vi "Resistance_measuremetn.vi"() -> ()   [LabVIEW 2015]
panel:
  out "XY Graph 2":cluster{dbl[], dbl[]}(graph)
  in  "Sample 2":refnum<visa-resource-name>
  out "number":dbl
  in  "milliseconds to wait":u32
  in  "VISA resource name 2":refnum<visa-resource-name>
  in  "Sample 1":refnum<visa-resource-name>
  in  "stop":bool
  out "XY Graph":cluster{dbl[], dbl[]}(graph)
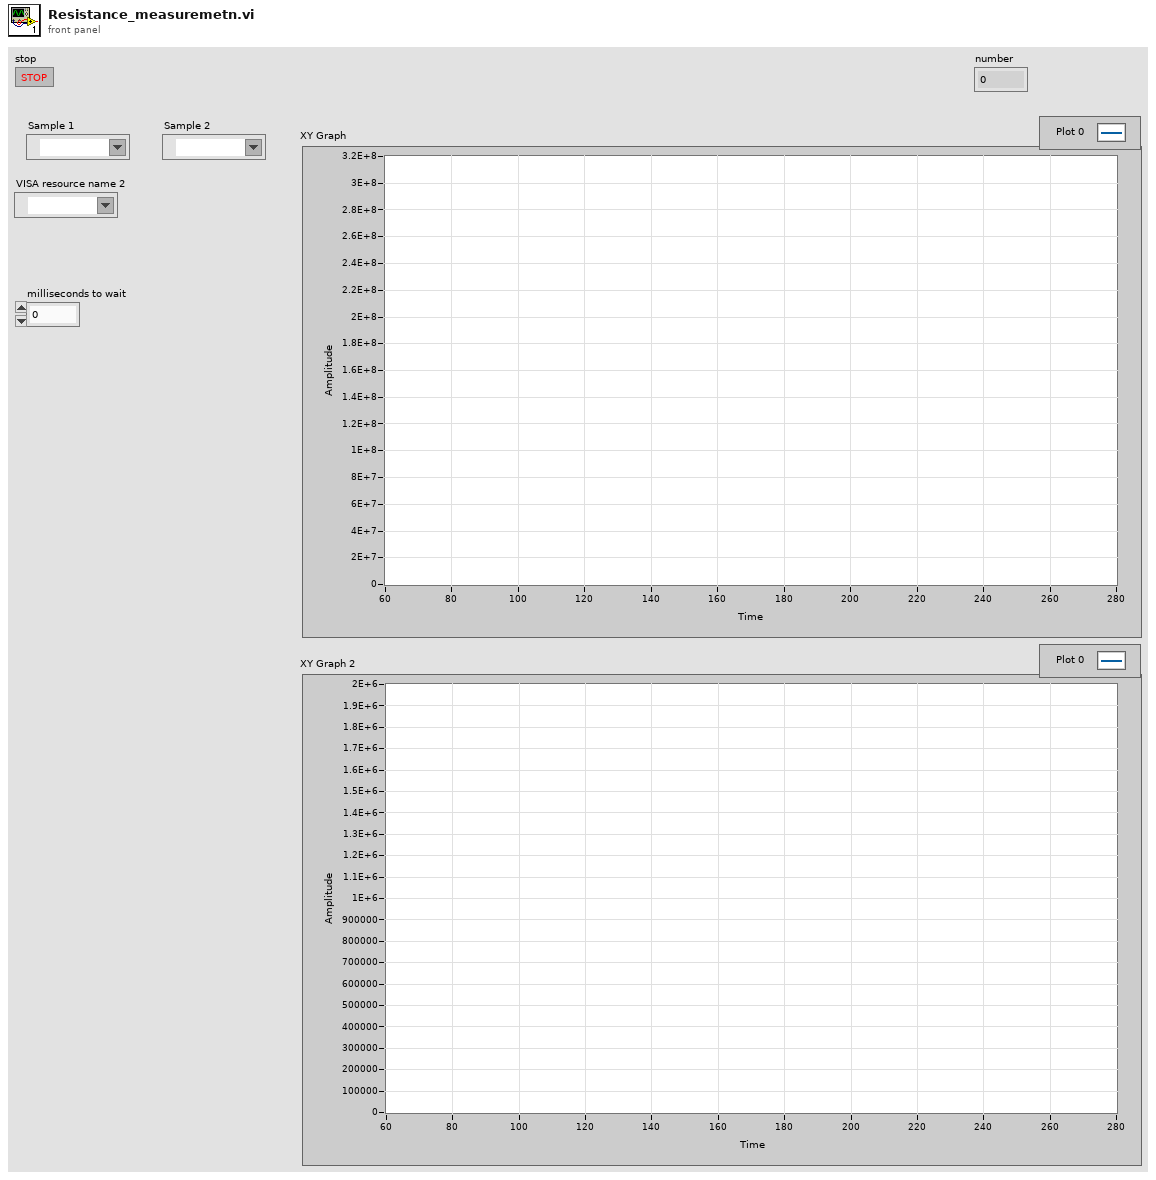
[diagram p1: front panel]
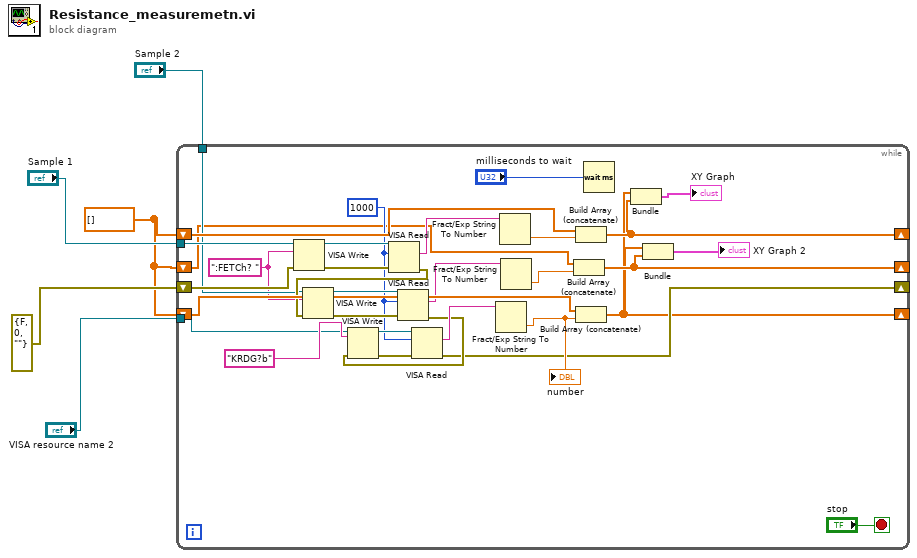
[diagram p0: block diagram]
diagram:
  w1 = dbl[] []
  n1 = while {
    tunnel: "Sample 1" -> [w35]
    tunnel: "VISA resource name 2" -> [w29]
    shift-right: [w7] -> _
    shift-left: w1 -> [w26]
    shift-right: [w23] -> _
    shift-left: w1 -> [w24]
    shift-right: [w17] -> _
    shift-left: errorcluster {"status"=FALSE, "code"=0, "source"=""} ("error out") -> [w16]
    tunnel: "Sample 2" -> [w15]
    shift-right: [w8] -> _
    shift-left: w1 -> [w9]
    stop <- "stop" stop-if-true
    w13 = ":FETCh? " ("write buffer")
    w12 = u32 1000 ("byte count")
    n2 = VISA Write(VISA resource name=w35, write buffer=w13, error in (no error)=w16) -> (VISA resource name out=w34:refnum<visa-resource-name>, error out=w36:errorcluster)  [unwired: 1 out]
    n3 = VISA Read(VISA resource name=w34, byte count=w12, error in (no error)=w36) -> (read buffer=w33:string, error out=w20:errorcluster)  [unwired: 2 out]
    n4 = VISA Write(VISA resource name=w15, write buffer=w13, error in (no error)=w20) -> (VISA resource name out=w14:refnum<visa-resource-name>, error out=w19:errorcluster)  [unwired: 1 out]
    n5 = VISA Read(VISA resource name=w14, byte count=w12, error in (no error)=w19) -> (read buffer=w11:string, error out=w18:errorcluster)  [unwired: 2 out]
    n6 = VISA Write(VISA resource name=w29, write buffer="KRDG?b", error in (no error)=w18) -> (VISA resource name out=w30:refnum<visa-resource-name>, error out=w32:errorcluster)  [unwired: 1 out]
    n7 = VISA Read(VISA resource name=w30, byte count=w12, error in (no error)=w32) -> (read buffer=w28:string, error out=w17:errorcluster)  [unwired: 2 out]
    n8 = Fract/Exp String To Number(string=w28) -> (number=w27:dbl)  [unwired: 3 in, 1 out]
    "number" <- w27
    n9 = Fract/Exp String To Number(string=w33) -> (number=w25:dbl)  [unwired: 3 in, 1 out]
    n10 = Fract/Exp String To Number(string=w11) -> (number=w10:dbl)  [unwired: 3 in, 1 out]
    n11 = Build Array (concatenate)(w9, w10) -> (w8:dbl[])
    n12 = Build Array (concatenate)(w24, w25) -> (w23:dbl[])
    n13 = Build Array (concatenate)(w26, w27) -> (w7:dbl[])
    n14 = Wait (ms)(milliseconds to wait="milliseconds to wait") -> ()  [unwired: 1 out]
    n15 = Bundle(w7, w23) -> (→"XY Graph":cluster{dbl[], dbl[]})  [unwired: 1 in]
    n16 = Bundle(w7, w8) -> (→"XY Graph 2":cluster{dbl[], dbl[]})  [unwired: 1 in]
  }
